vi "compare pkg versions server vs client.vi"(8 "error in (no error)":errorcluster) -> (0 "error out":errorcluster, 1 "Jl Server state out":T3, 2 "Pkg v LV client":T4, 3 "Pkg v Jl server":T4, 4 "return code":u8, 5 "timeout?":bool, 6 "detailed error info":T1)   [LabVIEW 2018, in "LV-0mq-Julia_roundtrip-lib.lvlib" / "LV2Julia_core.lvlib"]
uses:
  LV2Julia_core.lvlib
  VersionNumber.ctl
  Server or client state.ctl
  detailed error info.ctl
  StackFrame.ctl
  ef5b6aa2-77b9-48db-bc29-60677fa9782d.vi
  ef5b6aa2-77b9-48db-bc29-60677fa9782d.vi/fa696959-ff54-4df1-ad61-91f56aa676f9.vi
  ef5b6aa2-77b9-48db-bc29-60677fa9782d.vi/fa696959-ff54-4df1-ad61-91f56aa676f9.vi/e663d45c-8341-492a-8bfe-e5d15bc12b3e.vi
  ef5b6aa2-77b9-48db-bc29-60677fa9782d.vi/fa696959-ff54-4df1-ad61-91f56aa676f9.vi/ea400754-61ff-4591-9597-15a6c505c72f.vi
  ef5b6aa2-77b9-48db-bc29-60677fa9782d.vi/fa696959-ff54-4df1-ad61-91f56aa676f9.vi/e7b86073-ba51-4ee3-bd9e-f80a77227615.vi
  check ID validity.vi
  bindata_descr to JSON.vi
  check cluster field names.vi
  concat JSON.vi
  build request.vi
  REQ full lifecycle.vi
  Parse server response.vi
  log jl exceptions.vi
  version nos global.vi
  <vilib>/Utility/error.llb/Error Cluster From Error Code.vi
  <vilib>/ErrorRing/Error Ring.xnode
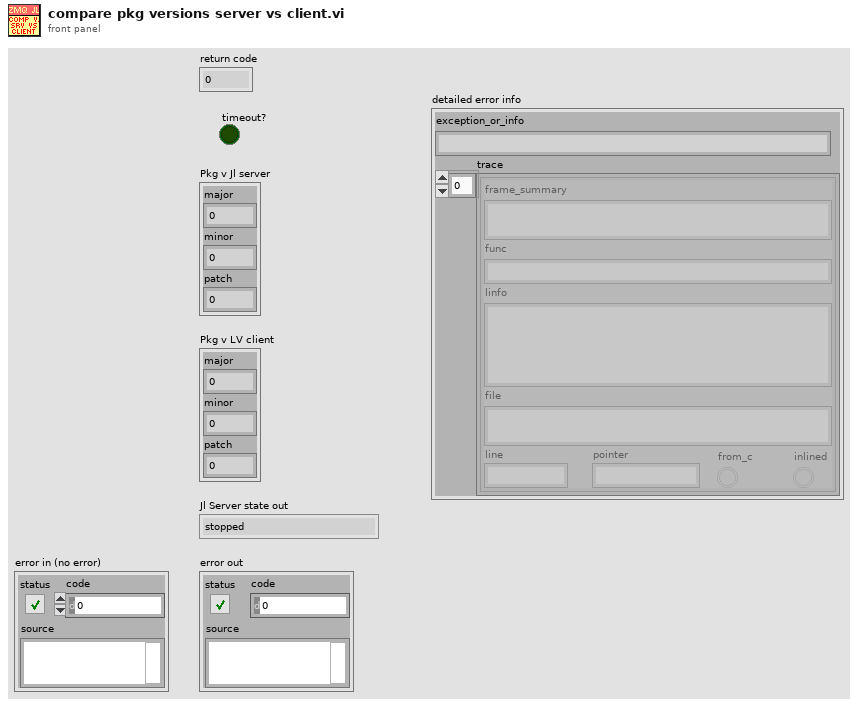
[diagram p1: front panel]
types:
  T1 = typedef "LV-0mq-Julia_roundtrip-lib.lvlib/LV2Julia_core.lvlib/detailed error info.ctl" = cluster{"exception_or_info":string, "trace":T2[]}
  T2 = typedef "LV-0mq-Julia_roundtrip-lib.lvlib/LV2Julia_core.lvlib/StackFrame.ctl" = cluster{"frame_summary":string, "func":string, "linfo":string, "file":string, "line":i32, "pointer":u64, "from_c":bool, "inlined":bool}
  T3 = typedef "LV-0mq-Julia_roundtrip-lib.lvlib/LV2Julia_core.lvlib/Server or client state.ctl" = enum16{"stopped", "running", "unknown"}
  T4 = typedef "LV-0mq-Julia_roundtrip-lib.lvlib/LV2Julia_core.lvlib/VersionNumber.ctl" = cluster{"major":u16, "minor":u16, "patch":u16}
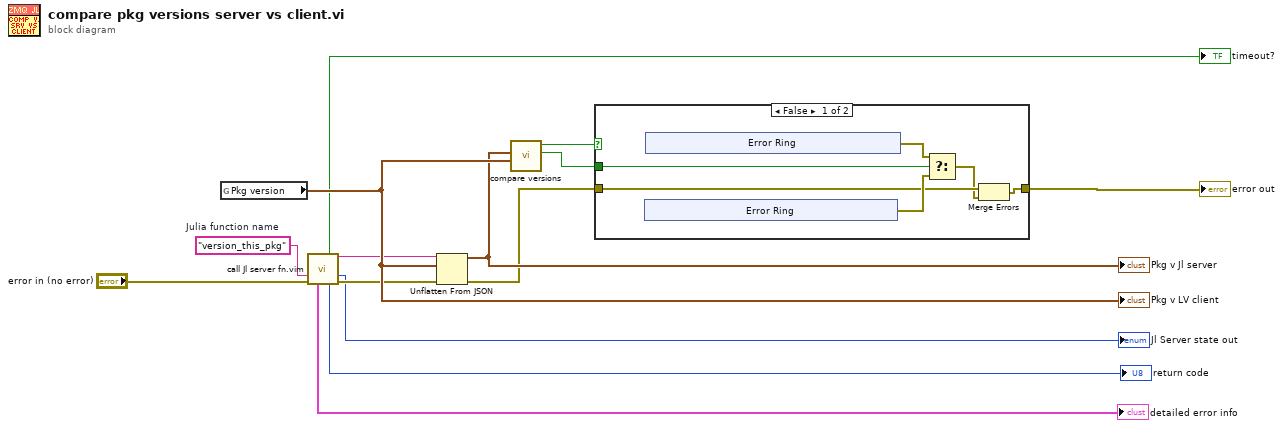
[diagram p0: block diagram]
diagram:
  w3 = "version_this_pkg"  # Julia function name
  n1 = global read "version nos global.vi" "Pkg version"() -> (w14:T4)
  "Pkg v LV client" <- w14
  n2 = call "call Jl server fn.vim"("fun2call"=w3, "error in (no error)"="error in (no error)") -> ("timeout?"=→"timeout?":bool, "JSON received"=w7:string, "Jl Server state out"=→"Jl Server state out":T3, "detailed error info"=→"detailed error info":T1, "return code"=→"return code":u8, "error out"=w6:errorcluster)  [unwired: 7 in, 1 out]
  n3 = Unflatten From JSON(JSON string=w7, type and defaults=w14, error in (no error)=w6) -> (value=w13:T4, error out=w10:errorcluster)  [unwired: 4 in]
  "Pkg v Jl server" <- w13
  n4 = call "compare versions.vi"("VersionNumber 2"=w14, "VersionNumber 1"=w13) -> ("1>2"=w12:bool, "1=2"=w9:bool)  [unwired: 7 in, 1 out]
  n5 = case shown="False" w9 {
    tunnel: w10 -> [w17 w31]
    tunnel: [w16 w31] -> w11
    tunnel: w12 -> [w20 _]
    frame False {
      n6 = xnode "Error Ring"() -> ("error out"=w18:errorcluster)
      n7 = xnode "Error Ring"() -> ("error out"=w19:errorcluster)
      n8 = Select(t=w19, s=w20, f=w18) -> (s? t:f=w15:errorcluster)
      n9 = Merge Errors(w17, w15) -> (w16:errorcluster)
    }
    frame True {
    }
  }
  "error out" <- w11
